vi "IsHotGoalPoly.vi"   [LabVIEW 2013]
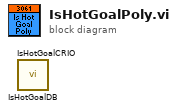
[diagram p0: block diagram]
diagram:
  n1 = call "IsHotGoalDB.vi"() -> ()  [unwired: 10 in, 2 out]
  n2 = call "IsHotGoalCRIO.vi"() -> ()  [unwired: 10 in, 2 out]
